vi "Get Launching VI Name.vi"(8 "error in (no error)":errorcluster, 11 "Search in":refnum<class "Search.lvclass">) -> (0 "error out":errorcluster, 2 "Launching VI Name":string, 3 "Search out":refnum<class "Search.lvclass">)   [LabVIEW 2020, in "Better Search.lvlib" / "Search.lvclass"]
uses:
  Search.lvclass
  Search.lvclass/Search.ctl
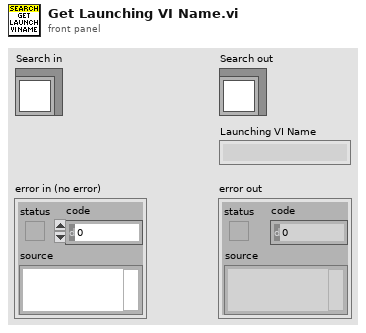
[diagram p1: front panel]
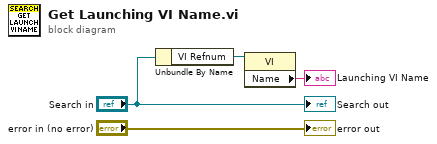
[diagram p0: block diagram]
diagram:
  n1 = Unbundle By Name("Search in") -> ("VI Refnum"=w2:refnum<vi>)
  n2 = property class="VI"(reference=w2) -> ("Name"=→"Launching VI Name":string)  [unwired: 1 in, 2 out]
  "error out" <- "error in (no error)"
  "Search out" <- "Search in"
